vi "increment file name.vi"(11 "file path in":path) -> (3 "incremented path":path)   [LabVIEW 2013]
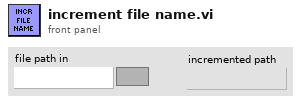
[diagram p1: front panel]
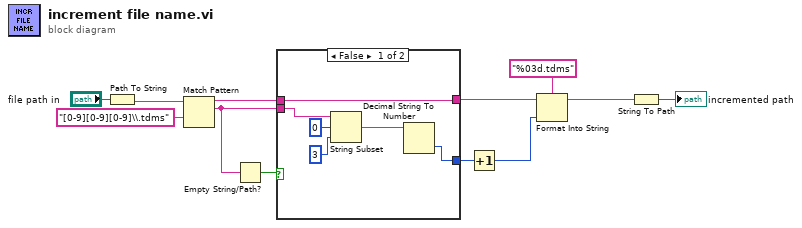
[diagram p0: block diagram]
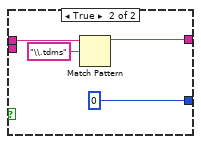
[diagram p2: hidden frame]
diagram:
  n1 = Path To String(path="file path in") -> (string=w12:string)
  n2 = Match Pattern(string=w12, regular expression="[0-9][0-9][0-9]\\.tdms") -> (before substring=w8:string, match substring=w7:string)  [unwired: 1 in, 2 out]
  n3 = Empty String/Path?(string/path=w7) -> (empty?=w9:bool)
  n4 = case shown="False" w9 {
    tunnel: w8 -> [w18 w22]
    tunnel: w7 -> [w17 _]
    tunnel: [w18 w20] -> w4
    tunnel: [w13 0] -> w6
    frame False {
      n5 = String Subset(string=w17, offset (0)=0, length (rest)=3 ("length (rest)")) -> (substring=w14:string)
      n6 = Decimal String To Number(string=w14) -> (number=w13:i32)  [unwired: 2 in, 1 out]
    }
    frame True {
      n7 = Match Pattern(string=w22, regular expression="\\.tdms") -> (before substring=w20:string)  [unwired: 1 in, 3 out]
    }
  }
  n8 = Increment(x=w6) -> (x+1=w2:i32)
  n9 = Format Into String(format string="%03d.tdms", initial string=w4, w2) -> (resulting string=w1:string)  [unwired: 1 in, 1 out]
  n10 = String To Path(string=w1) -> (path=→"incremented path":path)
